vi "parametric curve data.vi"(2 "Add outliers?":bool, 3 "Signal type":T1(ring)) -> (0 "Y":dbl[](array[numeric]), 1 "X":dbl[](array[numeric]))   [LabVIEW 2016]
doc: "This VI generates data of various signal types."
uses:
  <vilib>/Analysis/1siggen.llb/Ramp Pattern by Samples.vi
  <vilib>/Analysis/NI_AALBase.lvlib
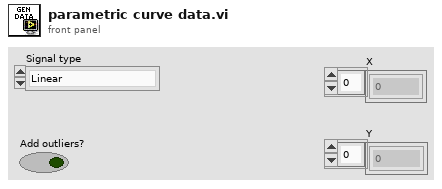
[diagram p1: front panel]
types:
  T1 = enum16{"Linear", "Exponential", "Power", "Gaussian", "Logarithmic"}
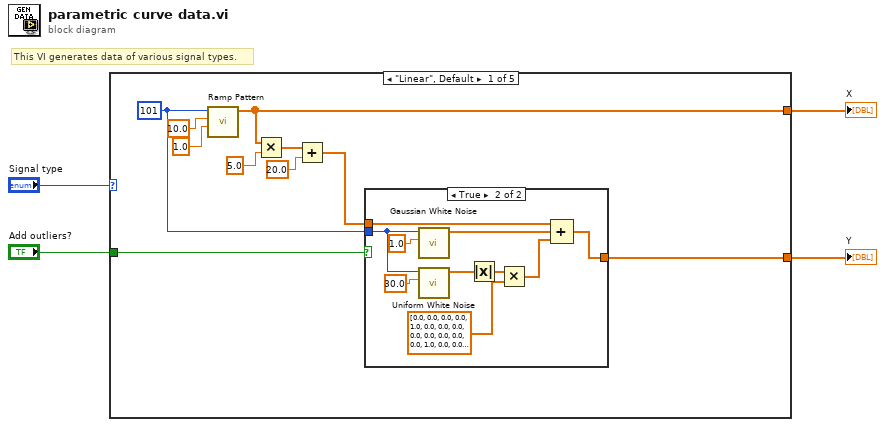
[diagram p0: block diagram]
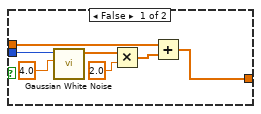
[diagram p2: hidden frame]
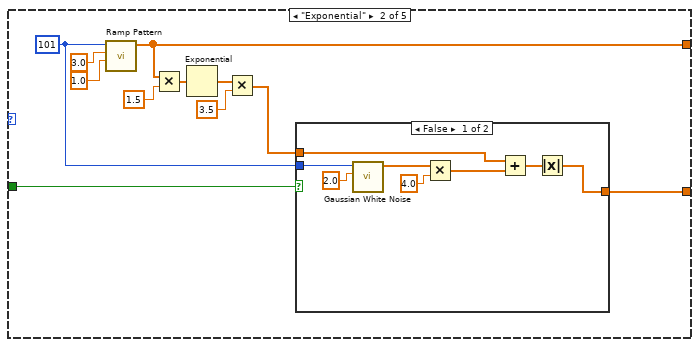
[diagram p3: hidden frame]
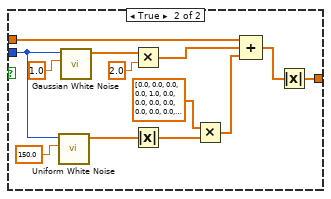
[diagram p4: hidden frame]
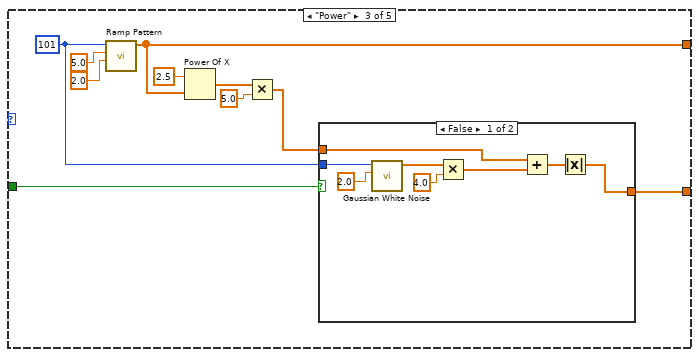
[diagram p5: hidden frame]
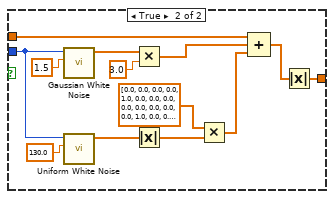
[diagram p6: hidden frame]
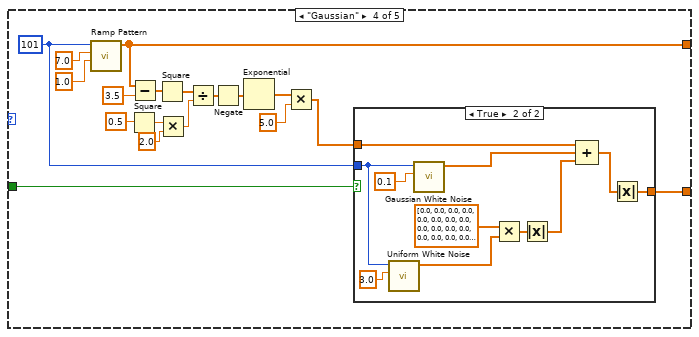
[diagram p7: hidden frame]
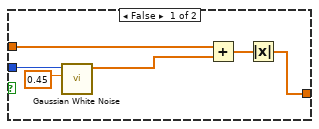
[diagram p8: hidden frame]
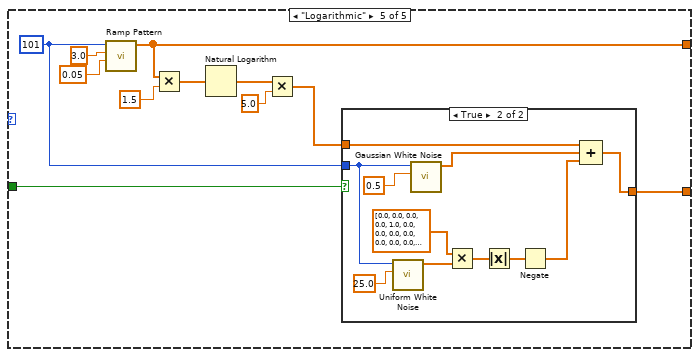
[diagram p9: hidden frame]
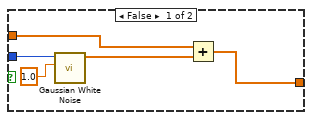
[diagram p10: hidden frame]
diagram:
  # "This VI generates data of various signal types."
  n1 = case shown="\"Linear\", Default" "Signal type" {
    tunnel: [w7 w37 w69 w109 w134] -> w3
    tunnel: [w12 w36 w66 w108 w133] -> w2
    tunnel: "Add outliers?" -> [w6 w38 w68 w110 w135]
    frame "Linear", Default {
      w5 = 101
      n2 = call-poly <vilib>:"Ramp Pattern.vi"("start"=1.0, "end"=10.0, "samples"=w5) -> ("Ramp Pattern"=w12:dbl[])  [unwired: 7 in, 1 out]
      n3 = Multiply(x=w12, y=5.0 ("start")) -> (x*y=w10:dbl[])
      n4 = Add(x=w10, y=20.0) -> (x+y=w8:dbl[])
      n5 = case shown="True" w6 {
        tunnel: w8 -> [w15 w30]
        tunnel: w5 -> [w21 w29]
        tunnel: [w16 w24] -> w7
        frame False {
          n6 = call <vilib>:"Gaussian White Noise.vi"("standard deviation"=4.0, "samples"=w21) -> ("Gaussian noise pattern"=w19:dbl[])  [unwired: 8 in, 1 out]
          n7 = Multiply(x=w19, y=2.0 ("standard deviation")) -> (x*y=w18:dbl[])
          n8 = Add(x=w15, y=w18) -> (x+y=w16:dbl[])
        }
        frame True {
          n9 = call <vilib>:"Gaussian White Noise.vi"("standard deviation"=1.0, "samples"=w29) -> ("Gaussian noise pattern"=w25:dbl[])  [unwired: 8 in, 1 out]
          n10 = call <vilib>:"Uniform White Noise.vi"("amplitude"=30.0, "samples"=w29) -> ("uniform white noise"=w22:dbl[])  [unwired: 8 in, 1 out]
          n11 = Absolute Value(x=w22) -> (abs(x)=w27:dbl[])
          n12 = Multiply(x=w27, y=dbl[] [0.0, 0.0, 0.0, 0.0, 1.0, 0.0, 0.0, 0.0, 0.0, 0.0, 0.0, 0.0, 0.0, 1.0, 0.0, 0.0, 0.0, 0.0, 0.0, 0.0, 0.0, 0.0, 0.0, 0.0, 0.0, 1.0, 0.0, 0.0, 0.0, 0.0, 0.0, 0.0, 0.0, 0.0, 0.0, 0.0, 0.0, 0.0, 0.0, 0.0, 1.0, 0.0, 0.0, 0.0, 0.0, 0.0, 0.0, 0.0, 0.0, 0.0, 0.0, 0.0, 0.0, 0.0, 0.0, 0.0, 0.0, 0.0, 0.0, 0.0, 0.0, -1.0, 0.0, 0.0, 0.0, 0.0, 0.0, 0.0, 0.0, 0.0, 0.0, 0.0, 0.0, 0.0, -1.0, 0.0, 0.0, 0.0, 0.0, 0.0, 0.0, 0.0, 0.0, 0.0, 0.0, 0.0, 0.0, -1.0, 0.0, 0.0, 0.0, 0.0, 0.0, 0.0, 0.0, 0.0, -1.0, 0.0, 0.0, 0.0, 0.0] ("x")) -> (x*y=w23:dbl[])
          n13 = Compound Arithmetic op=ADD(w30, w25, w23) -> (w24:dbl[])
        }
      }
    }
    frame "Exponential" {
      w39 = 101
      n14 = call-poly <vilib>:"Ramp Pattern.vi"("start"=1.0, "end"=3.0, "samples"=w39) -> ("Ramp Pattern"=w36:dbl[])  [unwired: 7 in, 1 out]
      n15 = Multiply(x=w36, y=1.5 ("start")) -> (x*y=w35:dbl[])
      n16 = Exponential(1:w35) -> (0:w33:dbl[])
      n17 = Multiply(x=w33, y=3.5) -> (x*y=w34:dbl[])
      n18 = case shown="False" w38 {
        tunnel: w34 -> [w43 w53]
        tunnel: w39 -> [w50 w59]
        tunnel: [w44 w54] -> w37
        frame False {
          n19 = call <vilib>:"Gaussian White Noise.vi"("standard deviation"=2.0, "samples"=w50) -> ("Gaussian noise pattern"=w48:dbl[])  [unwired: 8 in, 1 out]
          n20 = Multiply(x=w48, y=4.0 ("standard deviation")) -> (x*y=w47:dbl[])
          n21 = Add(x=w43, y=w47) -> (x+y=w45:dbl[])
          n22 = Absolute Value(x=w45) -> (abs(x)=w44:dbl[])
        }
        frame True {
          n23 = call <vilib>:"Uniform White Noise.vi"("amplitude"=150.0, "samples"=w59) -> ("uniform white noise"=w57:dbl[])  [unwired: 8 in, 1 out]
          n24 = call <vilib>:"Gaussian White Noise.vi"("standard deviation"=1.0, "samples"=w59) -> ("Gaussian noise pattern"=w61:dbl[])  [unwired: 8 in, 1 out]
          n25 = Multiply(x=w61, y=2.0 ("standard deviation")) -> (x*y=w62:dbl[])
          n26 = Absolute Value(x=w57) -> (abs(x)=w56:dbl[])
          n27 = Multiply(x=dbl[] [0.0, 0.0, 0.0, 0.0, 1.0, 0.0, 0.0, 0.0, 0.0, 0.0, 0.0, 0.0, 0.0, 1.0, 0.0, 0.0, 0.0, 0.0, 0.0, 0.0, 0.0, 0.0, 0.0, 0.0, 0.0, 1.0, 0.0, 0.0, 0.0, 0.0, 0.0, 0.0, 0.0, 0.0, 0.0, 0.0, 0.0, 0.0, 0.0, 0.0, 1.0, 0.0, 0.0, 0.0, 0.0, 0.0, 0.0, 0.0, 0.0, 0.0, 0.0, 0.0, 0.0, 0.0, 0.0, 0.0, 0.0, 0.0, 0.0, 0.0, 0.0, -1.0, 0.0, 0.0, 0.0, 0.0, 0.0, 0.0, 0.0, 0.0, 0.0, 0.0, 0.0, 0.0, -1.0, 0.0, 0.0, 0.0, 0.0, 0.0, 0.0, 0.0, 0.0, 0.0, 0.0, 0.0, 0.0, -1.0, 0.0, 0.0, 0.0, 0.0, 0.0, 0.0, 0.0, 0.0, -1.0, 0.0, 0.0, 0.0, 0.0], y=w56) -> (x*y=w52:dbl[])
          n28 = Compound Arithmetic op=ADD(w53, w62, w52) -> (w51:dbl[])
          n29 = Absolute Value(x=w51) -> (abs(x)=w54:dbl[])
        }
      }
    }
    frame "Power" {
      w70 = 101
      n30 = call-poly <vilib>:"Ramp Pattern.vi"("start"=2.0, "end"=5.0, "samples"=w70) -> ("Ramp Pattern"=w66:dbl[])  [unwired: 7 in, 1 out]
      n31 = Power Of X(1:w66, 2:2.5 ("start")) -> (0:w65:dbl[])
      n32 = Multiply(x=w65, y=5.0 ("start")) -> (x*y=w67:dbl[])
      n33 = case shown="False" w68 {
        tunnel: w67 -> [w74 w84]
        tunnel: w70 -> [w81 w90]
        tunnel: [w76 w85] -> w69
        frame False {
          n34 = call <vilib>:"Gaussian White Noise.vi"("standard deviation"=2.0, "samples"=w81) -> ("Gaussian noise pattern"=w79:dbl[])  [unwired: 8 in, 1 out]
          n35 = Multiply(x=w79, y=4.0 ("standard deviation")) -> (x*y=w78:dbl[])
          n36 = Add(x=w74, y=w78) -> (x+y=w75:dbl[])
          n37 = Absolute Value(x=w75) -> (abs(x)=w76:dbl[])
        }
        frame True {
          n38 = call <vilib>:"Gaussian White Noise.vi"("standard deviation"=1.5, "samples"=w90) -> ("Gaussian noise pattern"=w92:dbl[])  [unwired: 8 in, 1 out]
          n39 = call <vilib>:"Uniform White Noise.vi"("amplitude"=130.0, "samples"=w90) -> ("uniform white noise"=w88:dbl[])  [unwired: 8 in, 1 out]
          n40 = Multiply(x=w92, y=3.0 ("standard deviation")) -> (x*y=w93:dbl[])
          n41 = Absolute Value(x=w88) -> (abs(x)=w87:dbl[])
          n42 = Multiply(x=dbl[] [0.0, 0.0, 0.0, 0.0, 1.0, 0.0, 0.0, 0.0, 0.0, 0.0, 0.0, 0.0, 0.0, 1.0, 0.0, 0.0, 0.0, 0.0, 0.0, 0.0, 0.0, 0.0, 0.0, 0.0, 0.0, 1.0, 0.0, 0.0, 0.0, 0.0, 0.0, 0.0, 0.0, 0.0, 0.0, 0.0, 0.0, 0.0, 0.0, 0.0, 1.0, 0.0, 0.0, 0.0, 0.0, 0.0, 0.0, 0.0, 0.0, 0.0, 0.0, 0.0, 0.0, 0.0, 0.0, 0.0, 0.0, 0.0, 0.0, 0.0, 0.0, -1.0, 0.0, 0.0, 0.0, 0.0, 0.0, 0.0, 0.0, 0.0, 0.0, 0.0, 0.0, 0.0, -1.0, 0.0, 0.0, 0.0, 0.0, 0.0, 0.0, 0.0, 0.0, 0.0, 0.0, 0.0, 0.0, -1.0, 0.0, 0.0, 0.0, 0.0, 0.0, 0.0, 0.0, 0.0, -1.0, 0.0, 0.0, 0.0, 0.0], y=w87) -> (x*y=w82:dbl[])
          n43 = Compound Arithmetic op=ADD(w84, w93, w82) -> (w83:dbl[])
          n44 = Absolute Value(x=w83) -> (abs(x)=w85:dbl[])
        }
      }
    }
    frame "Gaussian" {
      w111 = 101
      n45 = call-poly <vilib>:"Ramp Pattern.vi"("start"=1.0, "end"=7.0, "samples"=w111) -> ("Ramp Pattern"=w108:dbl[])  [unwired: 7 in, 1 out]
      n46 = Square(x=0.5) -> (x^2=w101:dbl)
      n47 = Subtract(x=w108, y=3.5 ("start")) -> (x-y=w106:dbl[])
      n48 = Square(x=w106) -> (x^2=w105:dbl[])
      n49 = Multiply(x=w101, y=2.0) -> (x*y=w99:dbl)
      n50 = Divide(x=w105, y=w99) -> (x/y=w104:dbl[])
      n51 = Negate(x=w104) -> (-x=w103:dbl[])
      n52 = Exponential(1:w103) -> (0:w97:dbl[])
      n53 = Multiply(x=w97, y=5.0 ("start")) -> (x*y=w96:dbl[])
      n54 = case shown="True" w110 {
        tunnel: w96 -> [w113 w121]
        tunnel: w111 -> [w118 w128]
        tunnel: [w114 w122] -> w109
        frame False {
          n55 = call <vilib>:"Gaussian White Noise.vi"("standard deviation"=0.45, "samples"=w118) -> ("Gaussian noise pattern"=w116:dbl[])  [unwired: 8 in, 1 out]
          n56 = Add(x=w113, y=w116) -> (x+y=w115:dbl[])
          n57 = Absolute Value(x=w115) -> (abs(x)=w114:dbl[])
        }
        frame True {
          n58 = call <vilib>:"Uniform White Noise.vi"("amplitude"=3.0, "samples"=w128) -> ("uniform white noise"=w124:dbl[])  [unwired: 8 in, 1 out]
          n59 = call <vilib>:"Gaussian White Noise.vi"("standard deviation"=0.1, "samples"=w128) -> ("Gaussian noise pattern"=w125:dbl[])  [unwired: 8 in, 1 out]
          n60 = Multiply(x=dbl[] [0.0, 0.0, 0.0, 0.0, 0.0, 0.0, 0.0, 0.0, 0.0, 0.0, 0.0, 0.0, 0.0, 0.0, 0.0, 0.0, 0.0, 0.0, 0.0, 0.0, 1.0, 0.0, 0.0, 1.0, 0.0, 1.0, 1.0, 0.0, 0.0, 0.0, 1.0, 0.0, 0.0, 0.0, 0.0, 0.0, 0.0, 0.0, 0.0, 0.0, 0.0, 0.0, 0.0, 0.0, 0.0, 0.0, 0.0, 0.0, 0.0, 0.0, 0.0, 0.0, 0.0, 0.0, 1.0, 0.0, 0.0, 1.0, 0.0, 0.0, 1.0, 0.0, 0.0, 0.0, 0.0, 0.0, 0.0, 0.0, 0.0, 0.0, 0.0, 0.0, 0.0, 0.0, 0.0, 0.0, 0.0, 0.0, 0.0, 0.0, 0.0, 0.0, 0.0, 0.0, 0.0, 0.0, 0.0, 0.0, 0.0, 0.0, 0.0, 0.0, 0.0, 0.0, 0.0, 0.0, 0.0, 0.0, 0.0, 0.0, 0.0], y=w124) -> (x*y=w123:dbl[])
          n61 = Absolute Value(x=w123) -> (abs(x)=w119:dbl[])
          n62 = Compound Arithmetic op=ADD(w121, w125, w119) -> (w120:dbl[])
          n63 = Absolute Value(x=w120) -> (abs(x)=w122:dbl[])
        }
      }
    }
    frame "Logarithmic" {
      w136 = 101
      n64 = call-poly <vilib>:"Ramp Pattern.vi"("start"=0.05, "end"=3.0, "samples"=w136) -> ("Ramp Pattern"=w133:dbl[])  [unwired: 7 in, 1 out]
      n65 = Multiply(x=w133, y=1.5 ("start")) -> (x*y=w132:dbl[])
      n66 = Natural Logarithm(1:w132) -> (0:w131:dbl[])
      n67 = Multiply(x=w131, y=5.0) -> (x*y=w130:dbl[])
      n68 = case shown="True" w135 {
        tunnel: w130 -> [w141 w148]
        tunnel: w136 -> [w145 w155]
        tunnel: [w143 w147] -> w134
        frame False {
          n69 = call <vilib>:"Gaussian White Noise.vi"("standard deviation"=1.0, "samples"=w145) -> ("Gaussian noise pattern"=w142:dbl[])  [unwired: 8 in, 1 out]
          n70 = Add(x=w141, y=w142) -> (x+y=w143:dbl[])
        }
        frame True {
          n71 = call <vilib>:"Uniform White Noise.vi"("amplitude"=25.0, "samples"=w155) -> ("uniform white noise"=w151:dbl[])  [unwired: 8 in, 1 out]
          n72 = call <vilib>:"Gaussian White Noise.vi"("standard deviation"=0.5, "samples"=w155) -> ("Gaussian noise pattern"=w152:dbl[])  [unwired: 8 in, 1 out]
          n73 = Multiply(x=dbl[] [0.0, 0.0, 0.0, 0.0, 1.0, 0.0, 0.0, 0.0, 0.0, 0.0, 0.0, 0.0, 0.0, 1.0, 0.0, 0.0, 0.0, 0.0, 1.0, 0.0, 0.0, 0.0, 0.0, 0.0, 0.0, 1.0, 0.0, 0.0, 0.0, 0.0, 1.0, 0.0, 0.0, 0.0, 0.0, 0.0, 0.0, 0.0, 0.0, 0.0, 1.0, 0.0, 0.0, 0.0, 0.0, 0.0, 0.0, 0.0, 0.0, 0.0, 0.0, 1.0, 0.0, 0.0, 0.0, 0.0, 0.0, 0.0, 0.0, 0.0, 0.0, -1.0, 0.0, 0.0, 0.0, 0.0, 0.0, 0.0, 0.0, 0.0, 0.0, 0.0, 0.0, 0.0, -1.0, 0.0, 0.0, 0.0, 0.0, 0.0, 0.0, 0.0, 0.0, 0.0, 0.0, 0.0, 0.0, -1.0, 0.0, 0.0, 0.0, 0.0, 0.0, 0.0, 0.0, 0.0, -1.0, 0.0, 0.0, 0.0, 0.0], y=w151) -> (x*y=w150:dbl[])
          n74 = Absolute Value(x=w150) -> (abs(x)=w149:dbl[])
          n75 = Negate(x=w149) -> (-x=w146:dbl[])
          n76 = Compound Arithmetic op=ADD(w148, w152, w146) -> (w147:dbl[])
        }
      }
    }
  }
  "X" <- w2
  "Y" <- w3
